vi "Negotiate Server Connection.vi"(8 "error in (no error)":errorcluster, 11 "Client Controller in":refnum<class "Client Controller.lvclass">) -> (0 "error out":errorcluster, 3 "Client Controller out":refnum<class "Client Controller.lvclass">)   [LabVIEW 2026, in "Client Controller.lvlib" / "Client Controller.lvclass"]
uses:
  Client Controller.lvclass
  Client Controller.lvclass/Client Controller.ctl
  <vilib>/ErrorRing/Error Ring.xnode
  <vilib>/Utility/error.llb/Error Cluster From Error Code.vi
  <vilib>/ActorFramework/Stop Msg/Stop Msg.lvclass
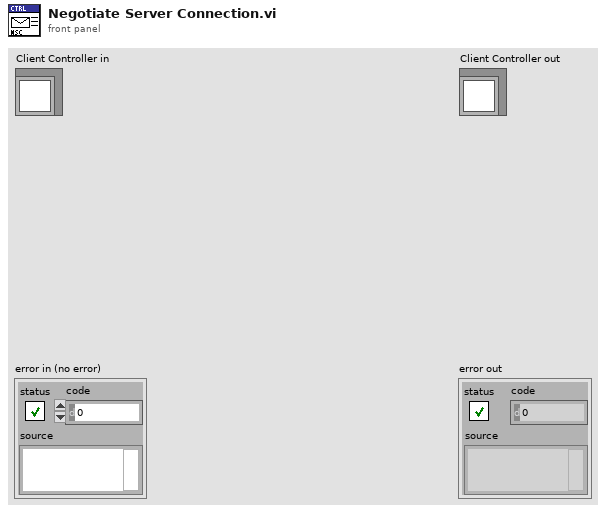
[diagram p1: front panel]
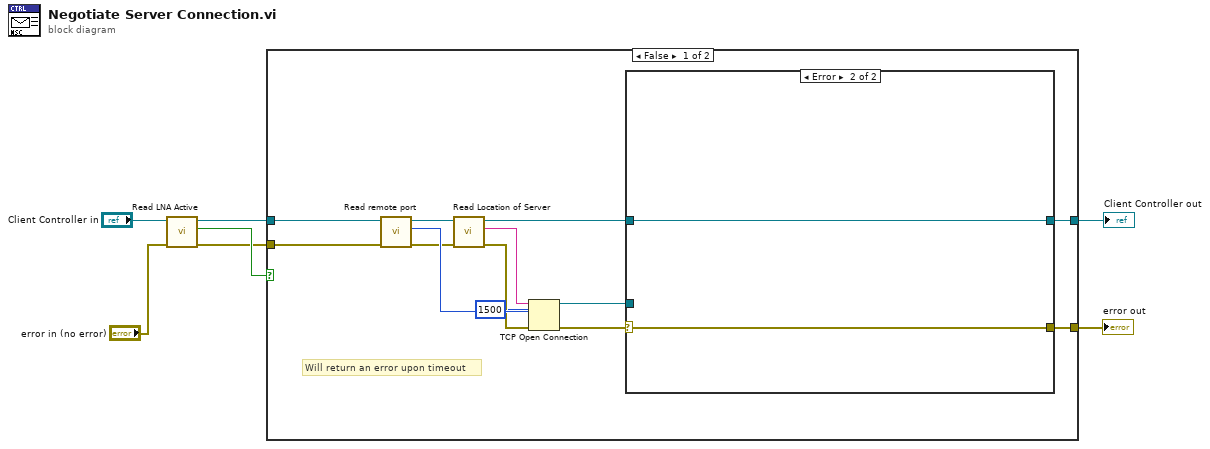
[diagram p0: block diagram]
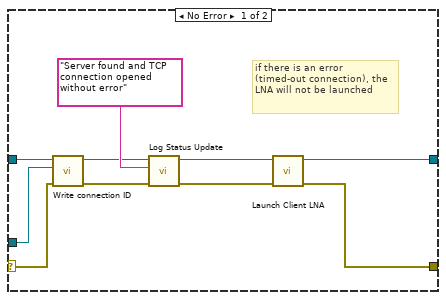
[diagram p2: hidden frame]
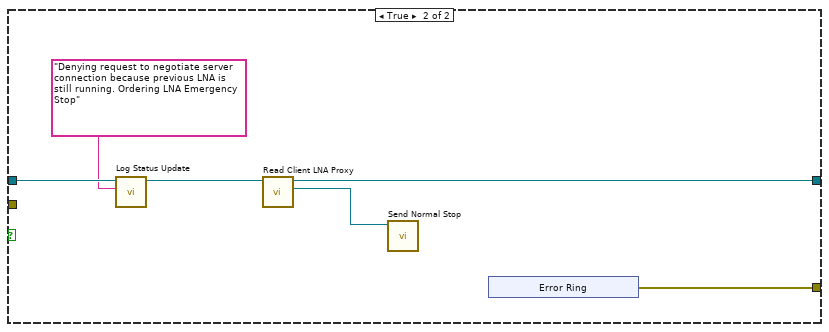
[diagram p3: hidden frame]
diagram:
  n1 = call "Read LNA Active.vi"("error in (no error)"="error in (no error)", "Client Controller in"="Client Controller in") -> ("error out"=w2:errorcluster, "LNA Active?"=w3:bool, "Client Controller out"=w4:refnum<class "Client Controller.lvclass">)  [unwired: 7 in]
  n2 = case shown="False" w3 {
    tunnel: w2 -> [w17 _]
    tunnel: [w11 w37] -> w7
    tunnel: [w10 w38] -> w6
    tunnel: w4 -> [w9 w36]
    frame False {
      # "Will return an error upon timeout"
      n3 = call "Read remote port.vi"("error in (no error)"=w17, "Client Controller in"=w9) -> ("error out"=w18:errorcluster, "remote port"=w19:u16, "Client Controller out"=w20:refnum<class "Client Controller.lvclass">)  [unwired: 7 in]
      n4 = call "Read Location of Server.vi"("error in (no error)"=w18, "Client Controller in"=w20) -> ("error out"=w13:errorcluster, "Location of Server"=w16:string, "Client Controller out"=w14:refnum<class "Client Controller.lvclass">)  [unwired: 7 in]
      n5 = TCP Open Connection(address=w16, remote port or service name=w19, timeout ms (60000)=1500, error in (no error)=w13) -> (connection ID=w15:refnum<k5>, error out=w12:errorcluster)  [unwired: 1 out]
      n6 = case shown="Error" w12 {
        selector: w12 -> [w25 w32]
        tunnel: w15 -> [w23 _]
        tunnel: w14 -> [w26 w31]
        tunnel: [w30 w31] -> w11
        tunnel: [w29 w32] -> w10
        frame No Error {
          # "if there is an error (timed-out connection), the\nLNA will not be launched"
          n7 = call "Write connection ID.vi"("error in (no error)"=w25, "connection ID"=w23, "Client Controller in"=w26) -> ("error out"=w22:errorcluster, "Client Controller out"=w24:refnum<class "Client Controller.lvclass">)  [unwired: 7 in]
          n8 = call-dynamic "Log Status Update.vi"("error in (no error)"=w22, "String"="Server found and TCP connection opened without error", "Controller in"=w24) -> ("error out"=w21:errorcluster, "Controller out"=w28:refnum<class "Client Controller.lvclass">)  [unwired: 7 in]
          n9 = call "Launch Client LNA.vi"("error in (no error)"=w21, "Client Controller in"=w28) -> ("error out"=w29:errorcluster, "Client Controller out"=w30:refnum<class "Client Controller.lvclass">)  [unwired: 8 in]
        }
        frame Error {
        }
      }
    }
    frame True {
      n10 = call-dynamic "Log Status Update.vi"("String"="Denying request to negotiate server connection because previous LNA is still running. Ordering LNA Emergency Stop", "Controller in"=w36) -> ("Controller out"=w35:refnum<class "Client Controller.lvclass">)  [unwired: 8 in, 1 out]
      n11 = call "Read Client LNA Proxy.vi"("Client Controller in"=w35) -> ("Actor Framework:Message Enqueuer"=w33:refnum<class "Message Enqueuer.lvclass">, "Client Controller out"=w37:refnum<class "Client Controller.lvclass">)  [unwired: 8 in, 1 out]
      n12 = call <vilib>:"Send Normal Stop.vi"("Message Enqueuer"=w33) -> ()  [unwired: 10 in, 1 out]
      n13 = xnode "Error Ring"() -> ("error out"=w38:errorcluster)
    }
  }
  "error out" <- w6
  "Client Controller out" <- w7
